vi "Create UI.vi"(8 "error in (no error)":errorcluster, 10 "instrument.PPMS.lvclass":refnum<class "instrument.PPMS.lvclass">, 11 "Instrument.PPMS UI in":refnum<class "Instrument.PPMS UI.lvclass">) -> (0 "error out":errorcluster, 3 "Instrument.PPMS UI out":refnum<class "Instrument.PPMS UI.lvclass">)   [LabVIEW 2016, in "Instrument.PPMS UI.lvclass"]
uses:
  Instrument.PPMS UI.lvclass
  instrument.PPMS/instrument.PPMS.lvclass
  Instrument.PPMS UI.lvclass/Instrument.PPMS UI.ctl
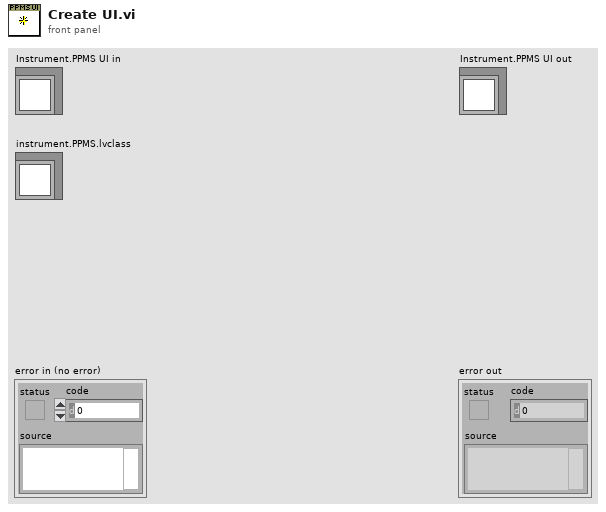
[diagram p1: front panel]
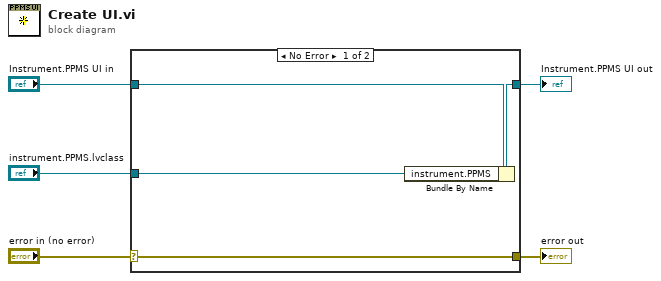
[diagram p0: block diagram]
diagram:
  n1 = case shown="No Error" "error in (no error)" {
    selector: "error in (no error)" -> [w9 w10]
    tunnel: [w9 w10] -> w4
    tunnel: [w7 w11] -> w2
    tunnel: "Instrument.PPMS UI in" -> [w8 w11]
    tunnel: "instrument.PPMS.lvclass" -> [w6 _]
    frame No Error {
      n2 = Bundle By Name(cluster=w8, "instrument.PPMS"=w6) -> (w7:refnum<class "Instrument.PPMS UI.lvclass">)
    }
    frame Error {
    }
  }
  "error out" <- w4
  "Instrument.PPMS UI out" <- w2
